vi "MouseDown.vi"(8 "error in":errorcluster, 9 "Coords":T1, 10 "ActTool":i32, 11 "reference":refnum<vi>) -> (0 "error out":errorcluster, 2 "StartPoints":cluster{i16, i16}[](array[cluster]))   [LabVIEW 2015, in "MyGraph.xctl"]
uses:
  MyGraph.xctl
  <vilib>/Utility/miscctls.llb/LVPoint32TypeDef.ctl
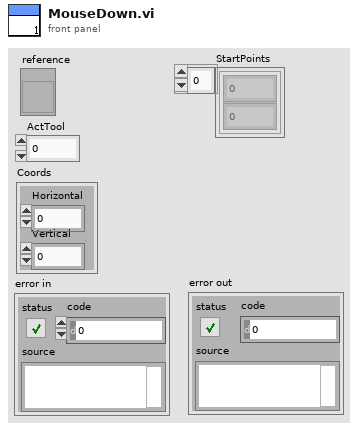
[diagram p1: front panel]
types:
  T1 = typedef "LVPoint32TypeDef.ctl" = cluster{"Horizontal":i32, "Vertical":i32}
  T2 = typedef "LVRectTypeDef.ctl" = cluster{"Left":i16, "Top":i16, "Right":i16, "Bottom":i16}
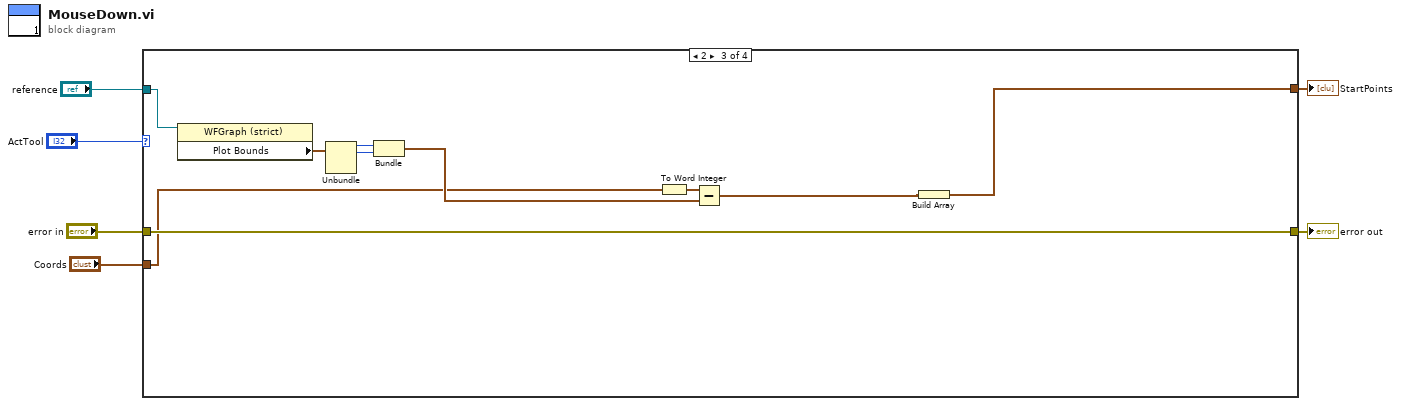
[diagram p0: block diagram]
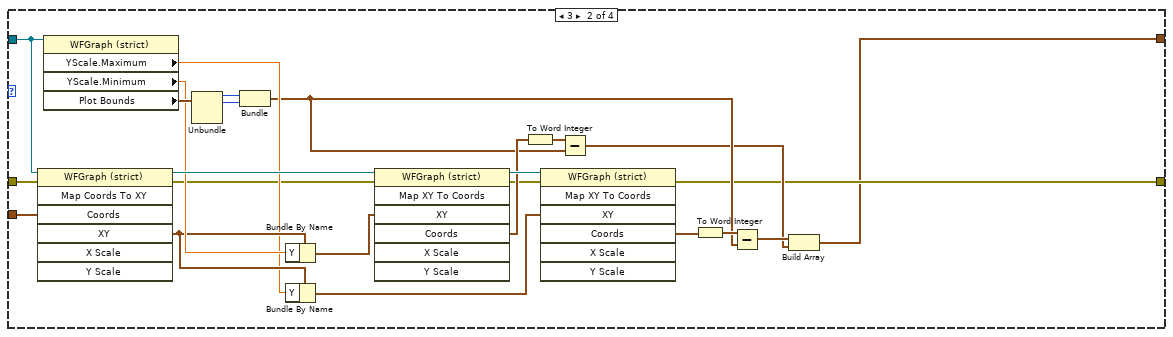
[diagram p3: hidden frame]
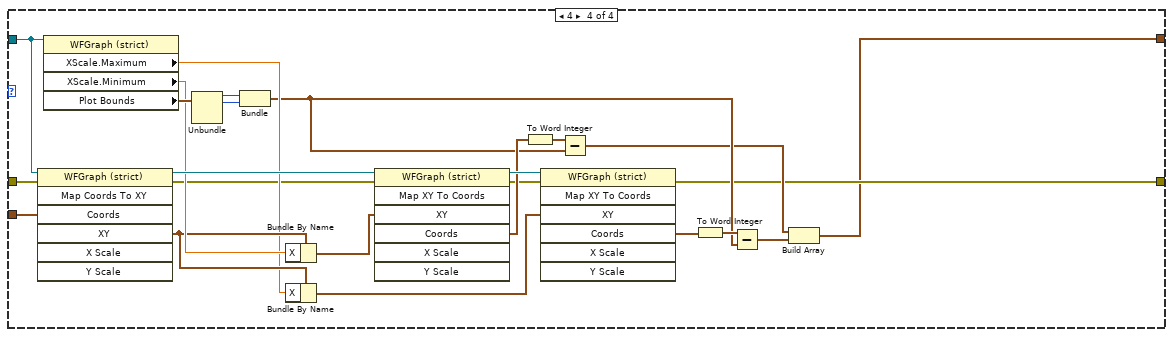
[diagram p4: hidden frame]
diagram:
  n1 = case shown="2" "ActTool" {
    tunnel: "Coords" -> [_ w13 w31 w47]
    tunnel: "reference" -> [_ w8 w33 w42]
    tunnel: [_ w10 w34 w44] -> w3
    tunnel: "error in" -> [_ w9 w34 w43]
    tunnel: [_ w7 w32 w41] -> w1
    frame 0, Default {
    }
    frame 3 {
      n2 = invoke class="WFGraph (strict)" method="Map Coords To XY"(reference=w8, error in=w9, "Coords"=w13) -> (reference out=w26:refnum<vi>, error out=w12:errorcluster, "XY"=w24:cluster{"X":dbl, "Y":dbl})  [unwired: 4 in, 4 out]
      n3 = property class="WFGraph (strict)"(reference=w8) -> ("YScale.Maximum"=w23:dbl, "YScale.Minimum"=w25:dbl, "Plot Bounds"=w30:T2)  [unwired: 1 in, 2 out]
      n4 = Unbundle(w30) -> ("Left"=w29:i16, "Top"=w28:i16)  [unwired: 2 out]
      n5 = Bundle("Left"=w29, "Top"=w28) -> (w16:cluster{"Left":i16, "Top":i16})  [unwired: 1 in]
      n6 = Bundle By Name(cluster=w24, "Y"=w25) -> (w22:cluster{"X":dbl, "Y":dbl})
      n7 = Bundle By Name(cluster=w24, "Y"=w23) -> (w20:cluster{"X":dbl, "Y":dbl})
      n8 = invoke class="WFGraph (strict)" method="Map XY To Coords"(reference=w26, error in=w12, "XY"=w22) -> (reference out=w21:refnum<vi>, error out=w11:errorcluster, "Coords"=w19:T1)  [unwired: 4 in, 4 out]
      n9 = To Word Integer(number=w19) -> (16bit integer=w27:cluster{"Horizontal":i16, "Vertical":i16})
      n10 = invoke class="WFGraph (strict)" method="Map XY To Coords"(reference=w21, error in=w11, "XY"=w20) -> (error out=w10:errorcluster, "Coords"=w18:T1)  [unwired: 4 in, 5 out]
      n11 = Subtract(x=w27, y=w16) -> (x-y=w14:cluster{i16, i16})
      n12 = To Word Integer(number=w18) -> (16bit integer=w17:cluster{"Horizontal":i16, "Vertical":i16})
      n13 = Subtract(x=w17, y=w16) -> (x-y=w15:cluster{i16, i16})
      n14 = Build Array(w15, w14) -> (w7:cluster{i16, i16}[])
    }
    frame 2 {
      n15 = property class="WFGraph (strict)"(reference=w33) -> ("Plot Bounds"=w40:T2)  [unwired: 1 in, 2 out]
      n16 = Unbundle(w40) -> ("Left"=w39:i16, "Top"=w38:i16)  [unwired: 2 out]
      n17 = Bundle("Left"=w39, "Top"=w38) -> (w36:cluster{"Left":i16, "Top":i16})  [unwired: 1 in]
      n18 = To Word Integer(number=w31) -> (16bit integer=w37:cluster{"Horizontal":i16, "Vertical":i16})
      n19 = Subtract(x=w37, y=w36) -> (x-y=w35:cluster{i16, i16})
      n20 = Build Array(w35) -> (w32:cluster{i16, i16}[])
    }
    frame 4 {
      n21 = invoke class="WFGraph (strict)" method="Map Coords To XY"(reference=w42, error in=w43, "Coords"=w47) -> (reference out=w60:refnum<vi>, error out=w46:errorcluster, "XY"=w58:cluster{"X":dbl, "Y":dbl})  [unwired: 4 in, 4 out]
      n22 = property class="WFGraph (strict)"(reference=w42) -> ("XScale.Maximum"=w57:dbl, "XScale.Minimum"=w59:dbl, "Plot Bounds"=w64:T2)  [unwired: 1 in, 2 out]
      n23 = Unbundle(w64) -> ("Left"=w63:i16, "Top"=w62:i16)  [unwired: 2 out]
      n24 = Bundle("Left"=w63, "Top"=w62) -> (w50:cluster{"Left":i16, "Top":i16})  [unwired: 1 in]
      n25 = Bundle By Name(cluster=w58, "X"=w59) -> (w56:cluster{"X":dbl, "Y":dbl})
      n26 = Bundle By Name(cluster=w58, "X"=w57) -> (w54:cluster{"X":dbl, "Y":dbl})
      n27 = invoke class="WFGraph (strict)" method="Map XY To Coords"(reference=w60, error in=w46, "XY"=w56) -> (reference out=w55:refnum<vi>, error out=w45:errorcluster, "Coords"=w53:T1)  [unwired: 4 in, 4 out]
      n28 = To Word Integer(number=w53) -> (16bit integer=w61:cluster{"Horizontal":i16, "Vertical":i16})
      n29 = invoke class="WFGraph (strict)" method="Map XY To Coords"(reference=w55, error in=w45, "XY"=w54) -> (error out=w44:errorcluster, "Coords"=w52:T1)  [unwired: 4 in, 5 out]
      n30 = Subtract(x=w61, y=w50) -> (x-y=w48:cluster{i16, i16})
      n31 = To Word Integer(number=w52) -> (16bit integer=w51:cluster{"Horizontal":i16, "Vertical":i16})
      n32 = Subtract(x=w51, y=w50) -> (x-y=w49:cluster{i16, i16})
      n33 = Build Array(w48, w49) -> (w41:cluster{i16, i16}[])
    }
  }
  "error out" <- w3
  "StartPoints" <- w1
